vi "Read Cluster.vi"(8 "error in (no error)":errorcluster, 11 "Grid in":refnum<class "Grid.lvclass">) -> (0 "error out":errorcluster, 2 "Cluster":T1, 3 "Grid out":refnum<class "Grid.lvclass">)   [LabVIEW 2016, in "Grid.lvclass"]
uses:
  Grid.lvclass
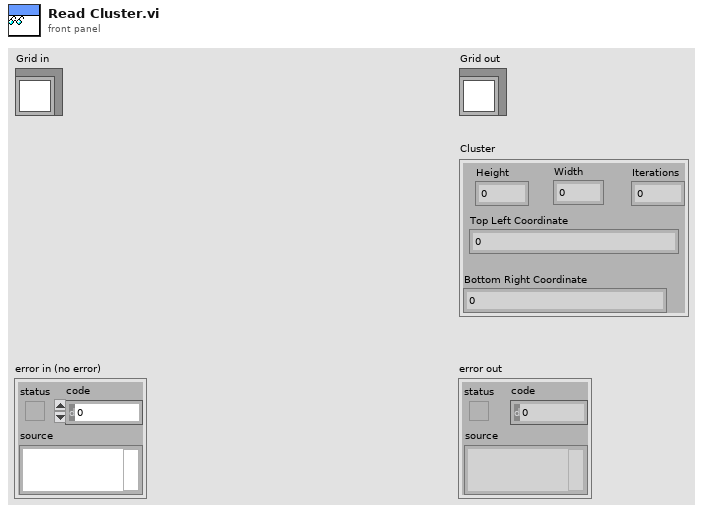
[diagram p1: front panel]
types:
  T1 = cluster{"Width":i32, "Height":i32, "Iterations":u16, "Top Left Coordinate":cdb, "Bottom Right Coordinate":cdb}
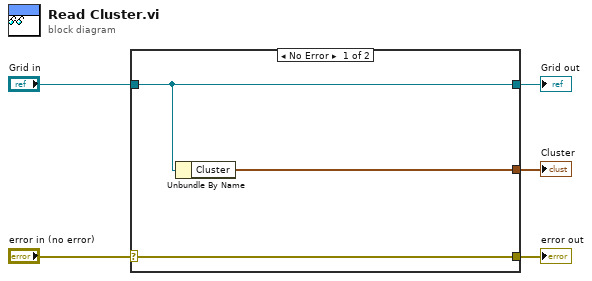
[diagram p0: block diagram]
diagram:
  n1 = case shown="No Error" "error in (no error)" {
    selector: "error in (no error)" -> [w8 w9]
    tunnel: [w8 w9] -> w4
    tunnel: [w7 w10] -> w2
    tunnel: "Grid in" -> [w7 w10]
    tunnel: [w6 _] -> w1
    frame No Error {
      n2 = Unbundle By Name(w7) -> ("Cluster"=w6:T1)
    }
    frame Error {
    }
  }
  "error out" <- w4
  "Grid out" <- w2
  "Cluster" <- w1
